vi "transmitter_LabVIEW.vi"() -> ()   [LabVIEW 2025]
uses:
  <vilib>/Instr/_visa.llb/VISA Configure Serial Port (Instr).vi
panel:
  in  "stop bits (10: 1 bit)":u16(ring)=10 items=["1.0"=10, "1.5"=15, "2.0"=20]
  in  "parity (0:none)":enum16{"None", "Odd", "Even", "Mark", "Space"}(ring)
  in  "data bits (8)":u16=8 min=5 max=8 step=1
  in  "baud rate (115200)":u32=9600
  out "Motor RPM":dbl[](array[numeric])
  out "Speed Chart":dbl[](graph)
  out "Status":string
  out "Mode":string
  out "Light Level":dbl
  out "Humidity (%)":dbl
  out "Temp (*C)":dbl
  in  "stop":bool
  in  "PID":bool
  in  "SetPoint":dbl
  in  "Stop":bool
  in  "Reverse":bool
  in  "Forward":bool
  in  "VISA COM Port":refnum<visa-resource-name>
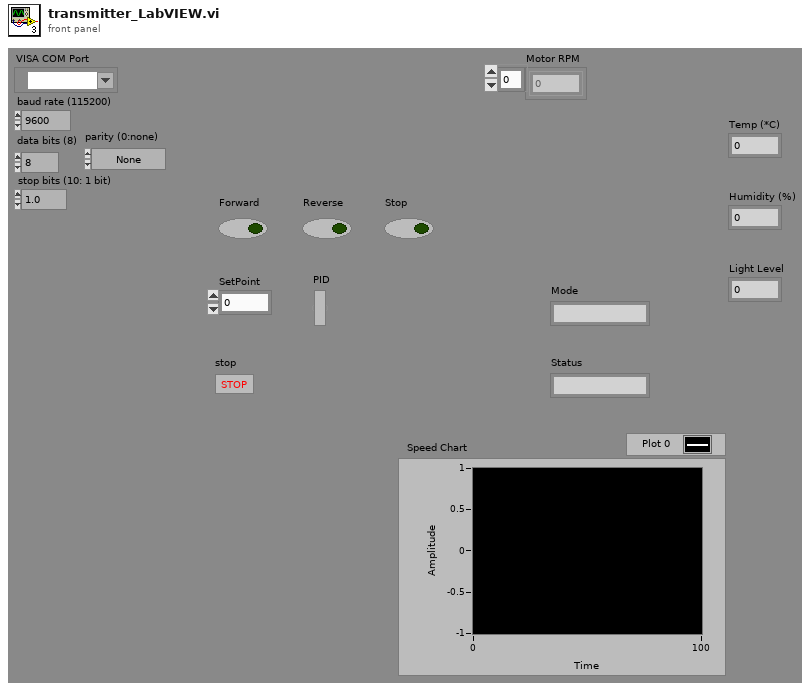
[diagram p1: front panel]
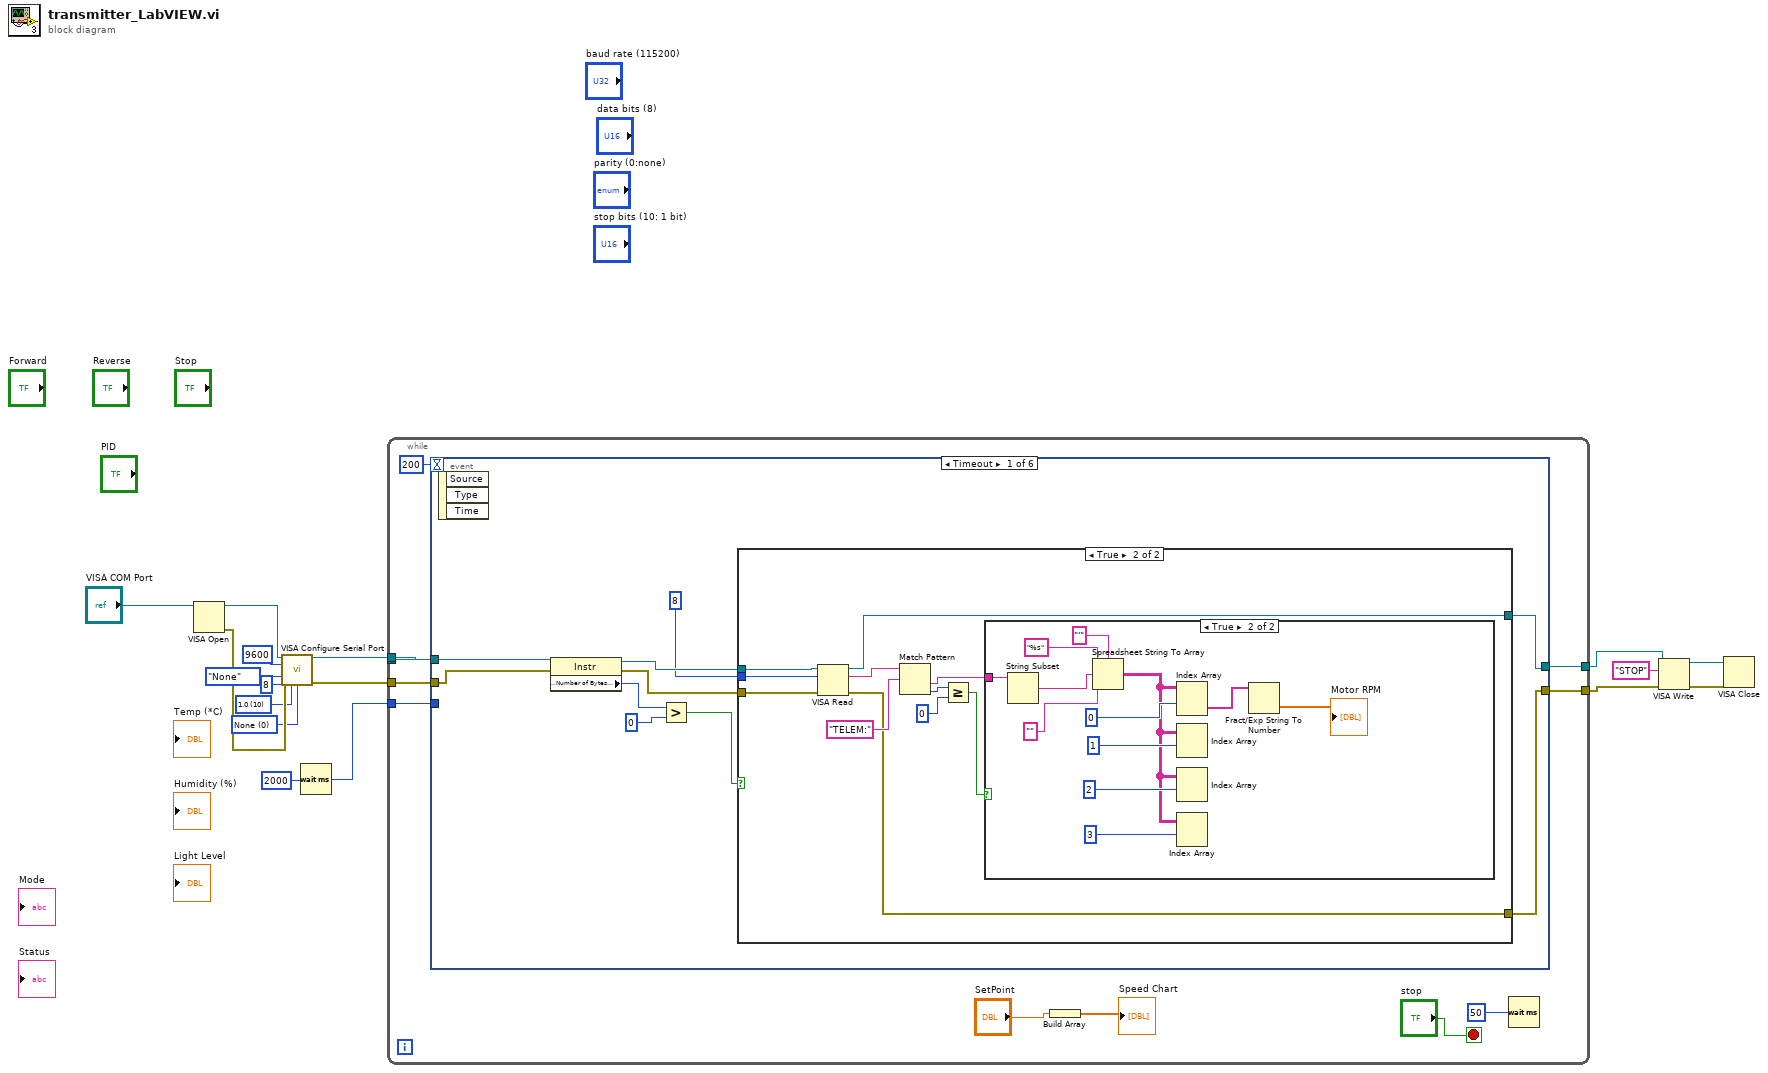
[diagram p0: block diagram]
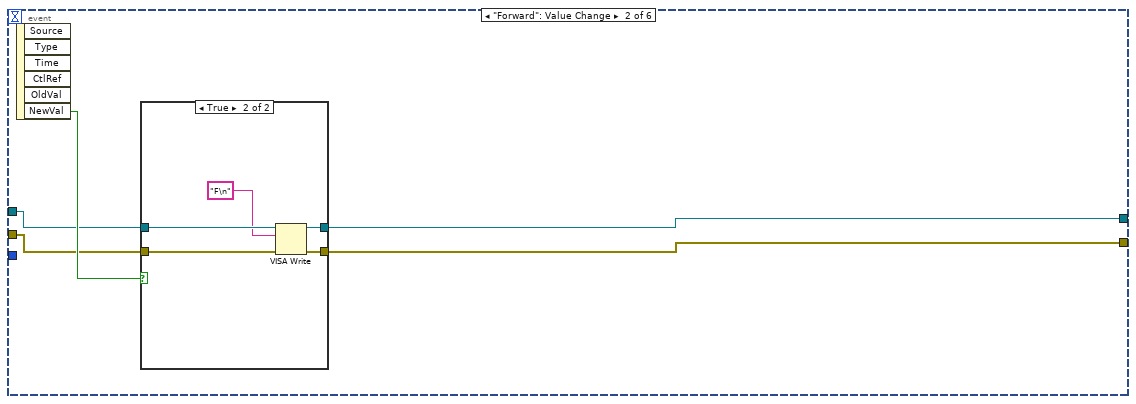
[diagram p4: hidden frame]
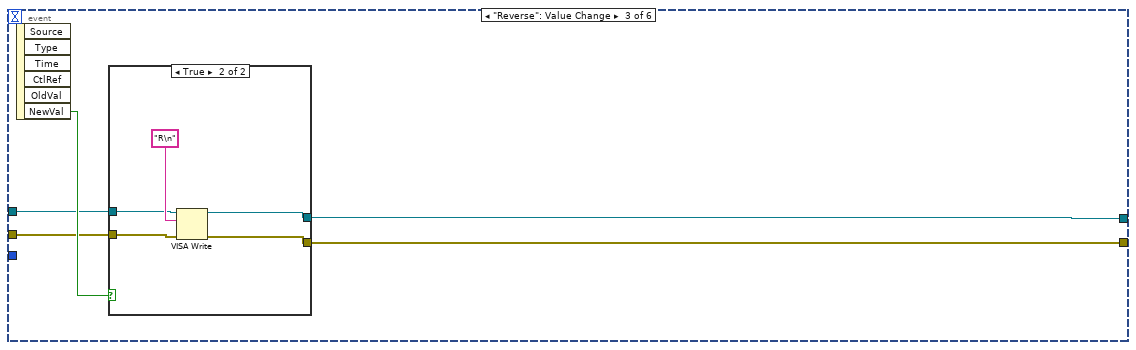
[diagram p6: hidden frame]
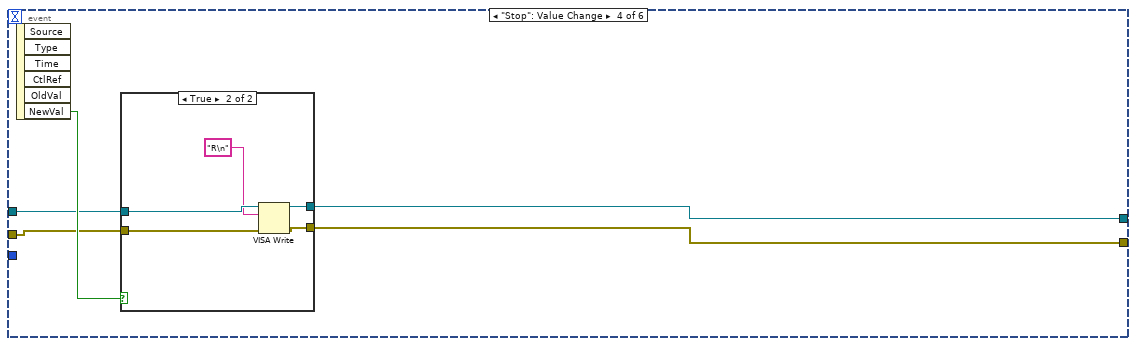
[diagram p8: hidden frame]
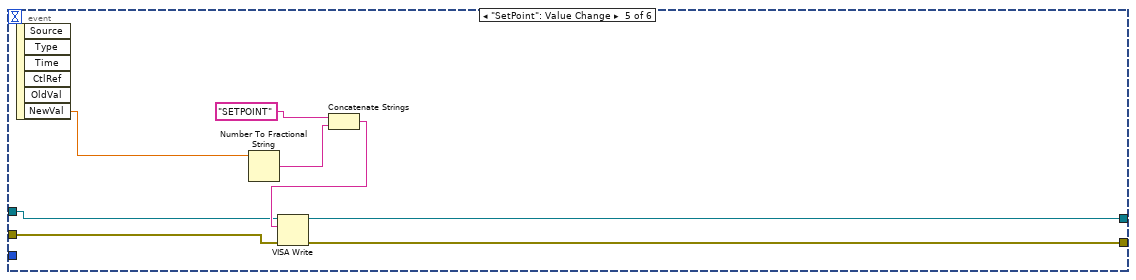
[diagram p10: hidden frame]
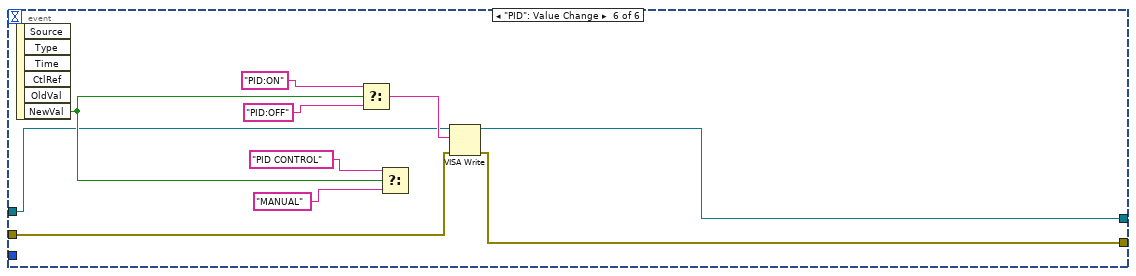
[diagram p11: hidden frame]
diagram:
  w10 = u16 0 items=["None", "XON/XOFF", "RTS/CTS", "XON/XOFF & RTS/CTS", "DTR/DSR", "XON/XOFF & DTR/DSR"] ("flow control (0:none)")
  w11 = u16 10 items=["1.0"=10, "1.5"=15, "2.0"=20] ("stop bits (10: 1 bit)")
  n1 = VISA Open(VISA resource name="VISA COM Port") -> (VISA resource name=w16:refnum<visa-resource-name>, error out=w15:errorcluster)  [unwired: 4 in]
  n2 = call-poly "VISA Configure Serial Port"("VISA resource name"=w16, "baud rate (9600)"=u32 9600, "data bits (8)"=u16 8, "parity (0:none)"=enum16{"None", "Odd", "Even", "Mark", "Space"}."None", "error in (no error)"=w15, "stop bits (10: 1 bit)"=w11, "flow control (0:none)"=w10) -> ("VISA resource name out"=w8:refnum<visa-resource-name>, "error out"=w7:errorcluster)  [unwired: 7 in]
  n3 = Wait (ms)(milliseconds to wait=u32 2000) -> (millisecond timer value=w6:u32)
  n4 = while {
    tunnel: [w26] -> _
    tunnel: w8 -> [w26]
    tunnel: w7 -> [w24]
    tunnel: w6 -> [w25]
    tunnel: [w22] -> w3
    tunnel: [w21] -> w4
    stop <- "stop" stop-if-true
    n5 = event shown="[0] Timeout" {
      selector: _ -> [_ _ _ _ _ _]
      dyn-events: _ -> [_ _ _ _ _ _]
      timeout: 200 -> [_ _ _ _ _ _]
      tunnel: w26 -> [w37 w66 w77 w90 w102 w110]
      tunnel: w25 -> [_ _ _ _ _ _]
      tunnel: w24 -> [w36 w65 w78 w89 w101 w109]
      tunnel: [w31 w64 w75 w88 w100 w108] -> w22
      tunnel: [w32 w63 w76 w87 w99 w107] -> w21
      event Timeout {
        n6 = event-data() -> ()  [unwired: 1 in, 3 out]
        n7 = property class="Instr"(reference=w37, error in=w36) -> (reference out=w34:refnum<visa-resource-name>, error out=w33:errorcluster, "Serial Settings:Number of Bytes at Serial Port"=w30:u32)
        n8 = Greater?(x=w30, y=u32 0) -> (0:w35:bool)
        n9 = case shown="True" w35 {
          tunnel: w34 -> [w39 w50]
          tunnel: w33 -> [w38 w49]
          tunnel: [w38 w47] -> w32
          tunnel: [w39 w46] -> w31
          tunnel: u32 8 ("byte count") -> [_ w40]
          frame False {
          }
          frame True {
            n10 = VISA Read(VISA resource name=w50, byte count=w40, error in (no error)=w49) -> (VISA resource name out=w46:refnum<visa-resource-name>, read buffer=w45:string, error out=w47:errorcluster)  [unwired: 1 out]
            n11 = Match Pattern(string=w45, regular expression="TELEM:") -> (after substring=w41:string, offset past match=w44:i32)  [unwired: 1 in, 2 out]
            n12 = Greater Or Equal?(x=w44, y=0) -> (x >= y?=w42:bool)
            n13 = case shown="True" w42 {
              tunnel: w41 -> [_ w58]
              frame False {
              }
              frame True {
                n14 = String Subset(string=w58) -> (substring=w56:string)  [unwired: 2 in]
                n15 = Spreadsheet String To Array(delimiter (Tab)="'", format string="%s", spreadsheet string=w56, array type (2D Dbl)="") -> (array=w53:string[][])
                n16 = Index Array "Index Array"(array=w53, index (row)=0) -> (element=w52:string[])  [unwired: 1 in]
                n17 = Index Array(array=w53, index (row)=1) -> ()  [unwired: 1 in, 1 out]
                n18 = Index Array(array=w53, index (row)=2) -> ()  [unwired: 1 in, 1 out]
                n19 = Index Array(array=w53, index (row)=3) -> ()  [unwired: 1 in, 1 out]
                n20 = Fract/Exp String To Number(string=w52) -> (number=→"Motor RPM":dbl[])  [unwired: 3 in, 1 out]
              }
            }
          }
        }
      }
      event "Forward": Value Change {
        n21 = event-data() -> ("NewVal"=w67:bool)  [unwired: 1 in, 5 out]
        n22 = case shown="True" w67 {
          tunnel: w66 -> [w68 w74]
          tunnel: w65 -> [w69 w73]
          tunnel: [w68 w71] -> w64
          tunnel: [w69 w70] -> w63
          frame False {
          }
          frame True {
            n23 = VISA Write(VISA resource name=w74, write buffer="F\n", error in (no error)=w73) -> (VISA resource name out=w71:refnum<visa-resource-name>, error out=w70:errorcluster)  [unwired: 1 out]
          }
        }
      }
      event "Reverse": Value Change {
        n24 = event-data() -> ("NewVal"=w79:bool)  [unwired: 1 in, 5 out]
        n25 = case shown="True" w79 {
          tunnel: w78 -> [w80 w85]
          tunnel: w77 -> [w81 w84]
          tunnel: [w81 w83] -> w75
          tunnel: [w80 w82] -> w76
          frame False {
          }
          frame True {
            n26 = VISA Write(VISA resource name=w84, write buffer="R\n", error in (no error)=w85) -> (VISA resource name out=w83:refnum<visa-resource-name>, error out=w82:errorcluster)  [unwired: 1 out]
          }
        }
      }
      event "Stop": Value Change {
        n27 = event-data() -> ("NewVal"=w91:bool)  [unwired: 1 in, 5 out]
        n28 = case shown="True" w91 {
          tunnel: w90 -> [w93 w98]
          tunnel: w89 -> [w92 w97]
          tunnel: [w93 w95] -> w88
          tunnel: [w92 w94] -> w87
          frame False {
          }
          frame True {
            n29 = VISA Write(VISA resource name=w98, write buffer="R\n", error in (no error)=w97) -> (VISA resource name out=w95:refnum<visa-resource-name>, error out=w94:errorcluster)  [unwired: 1 out]
          }
        }
      }
      event "SetPoint": Value Change {
        n30 = event-data() -> ("NewVal"=w106:dbl)  [unwired: 1 in, 5 out]
        n31 = Number To Fractional String(number=w106) -> (F-format string=w104:string)  [unwired: 3 in]
        n32 = Concatenate Strings("SETPOINT" ("F-format string"), w104) -> (w103:string)
        n33 = VISA Write(VISA resource name=w102, write buffer=w103, error in (no error)=w101) -> (VISA resource name out=w100:refnum<visa-resource-name>, error out=w99:errorcluster)  [unwired: 1 out]
      }
      event "PID": Value Change {
        n34 = event-data() -> ("NewVal"=w114:bool)  [unwired: 1 in, 5 out]
        n35 = Select(t="PID:ON", s=w114, f="PID:OFF") -> (s? t:f=w111:string)
        n36 = Select(t="PID CONTROL", s=w114, f="MANUAL") -> ()  [unwired: 1 out]
        n37 = VISA Write(VISA resource name=w110, write buffer=w111, error in (no error)=w109) -> (VISA resource name out=w108:refnum<visa-resource-name>, error out=w107:errorcluster)  [unwired: 1 out]
      }
    }
    n38 = Build Array("SetPoint") -> (→"Speed Chart":dbl[])
    n39 = Wait (ms)(milliseconds to wait=50) -> ()  [unwired: 1 out]
  }
  n40 = VISA Write(VISA resource name=w3, write buffer="STOP", error in (no error)=w4) -> (VISA resource name out=w1:refnum<visa-resource-name>, error out=w2:errorcluster)  [unwired: 1 out]
  n41 = VISA Close(VISA resource name=w1, error in (no error)=w2) -> ()  [unwired: 1 out]
